vi "Cache-GlobalEventRef.vi"(6 "Create? (F)":bool, 8 "error in (no error)":errorcluster) -> (0 "error out":errorcluster, 3 "Event":refnum<user-event>)   [LabVIEW 2017, in "Communicable State Machine.lvlib"]
doc: "-- <b>Controls</b> --\n- <b>Create(F)</b>:\n\n-- <b>Indicators</b> --\n- <b>CSM Global Log Event</b>:"
uses:
  Communicable State Machine.lvlib
  Typedef/_CSM_GlobalLog_MSG.ctl
  Typedef/_CSM_Response Source Message.ctl
  Typedef/_CSM_GlobalLog_MSG_TYPE.ctl
  ChangeFlag/ChangeFlag-Write.vi
  Utility/Random Change Flag.vi
  ChangeFlag/ChangeFlagDB.vi
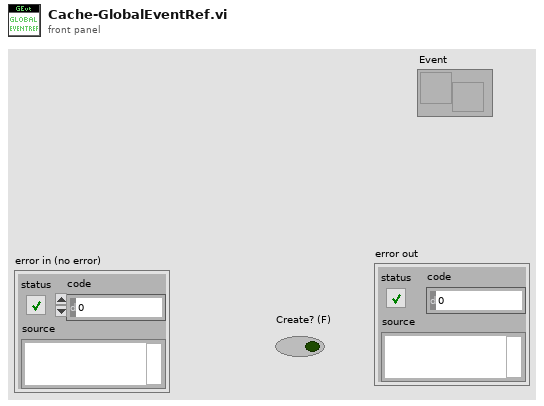
[diagram p1: front panel]
types:
  T1 = typedef "Communicable State Machine.lvlib/_CSM_GlobalLog_MSG.ctl" = cluster{"Name (\"\" to Use UUID)":string, "Current State":string, "Arguments":string, "Source Message":T2, "Source Module":string, "Complete(T)/Start(F)":bool, "LogType":T3, "Time Stamp":timestamp}
  T2 = typedef "Communicable State Machine.lvlib/_CSM_Response Source Message.ctl" = cluster{"‘State":string, "’Arguments":string, "’Error":errorcluster}
  T3 = typedef "Communicable State Machine.lvlib/_CSM_GlobalLog_MSG_TYPE.ctl" = enum16{"User Log", "State Change", "Status", "Interrupt", "Register", "Unregister", "Error Log", "Module Created", "Module Destroyed"}
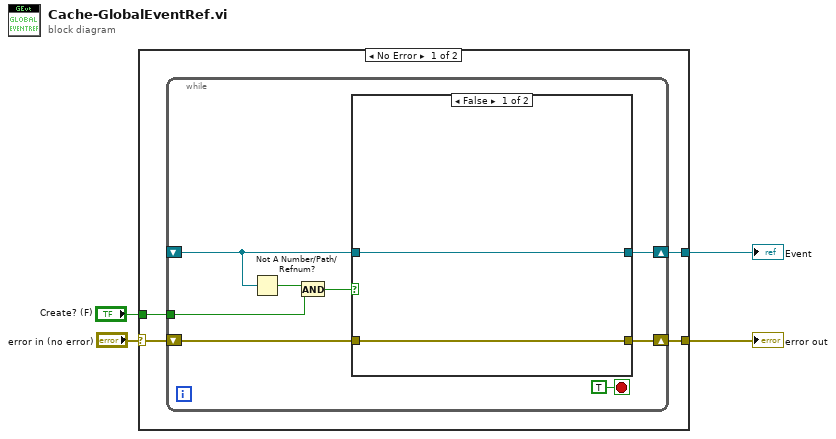
[diagram p0: block diagram]
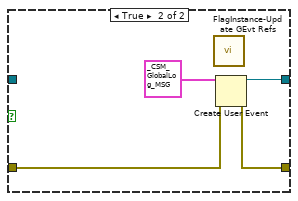
[diagram p2: hidden frame]
diagram:
  n1 = case shown="No Error" "error in (no error)" {
    selector: "error in (no error)" -> [w7 w23]
    tunnel: [w8 _] -> w4
    tunnel: [w6 w23] -> w2
    tunnel: "Create? (F)" -> [w5 _]
    frame No Error {
      n2 = while {
        shift-right: [w14] -> w6
        shift-left: w7 -> [w15]
        shift-right: [w16] -> w8
        shift-left: _ -> [w12]
        tunnel: w5 -> [w9]
        stop <- TRUE stop-if-true
        n3 = Not A Number/Path/Refnum?(number/path/refnum=w12) -> (NaN/Path/Refnum?=w10:bool)
        n4 = And(x=w10, y=w9) -> (x .and. y?=w11:bool)
        n5 = case shown="False" w11 {
          tunnel: [w18 w22] -> w16
          tunnel: w15 -> [w17 w20]
          tunnel: [w17 w21] -> w14
          tunnel: w12 -> [w18 _]
          frame False {
          }
          frame True {
            n6 = call "FlagInstance-Update GEvt Refs.vi"() -> ()  [unwired: 10 in, 2 out]
            n7 = Create User Event(user event datatype=T1 {"Name (\"\" to Use UUID)"="", "Current State"="", "Arguments"="", "Source Message"={"‘State"="", "’Arguments"="", "’Error"={"status"=FALSE, "code"=0, "source"=""}}, "Source Module"="", "Complete(T)/Start(F)"=FALSE, "LogType"=enum."State Change", "Time Stamp"=timestamp(0 s since 1904-01-01)} ("Cross JKI State Machine Data"), error in=w20) -> (user event=w22:refnum<user-event>, error out=w21:errorcluster)
          }
        }
      }
    }
    frame Error {
    }
  }
  "Event" <- w4
  "error out" <- w2
